vi "DrawStringOnFrontImage.vi"(6 "color(black)":u32(colorbox), 8 "error in":errorcluster, 10 "input string":string, 11 "Graph Ref":refnum<vi>) -> (0 "error out":errorcluster, 2 "picture out":picture)   [LabVIEW 2023]
doc: "Draws an Image according to input string and sets it as the Graph's front image."
uses:
  StringFormatGlobals.vi
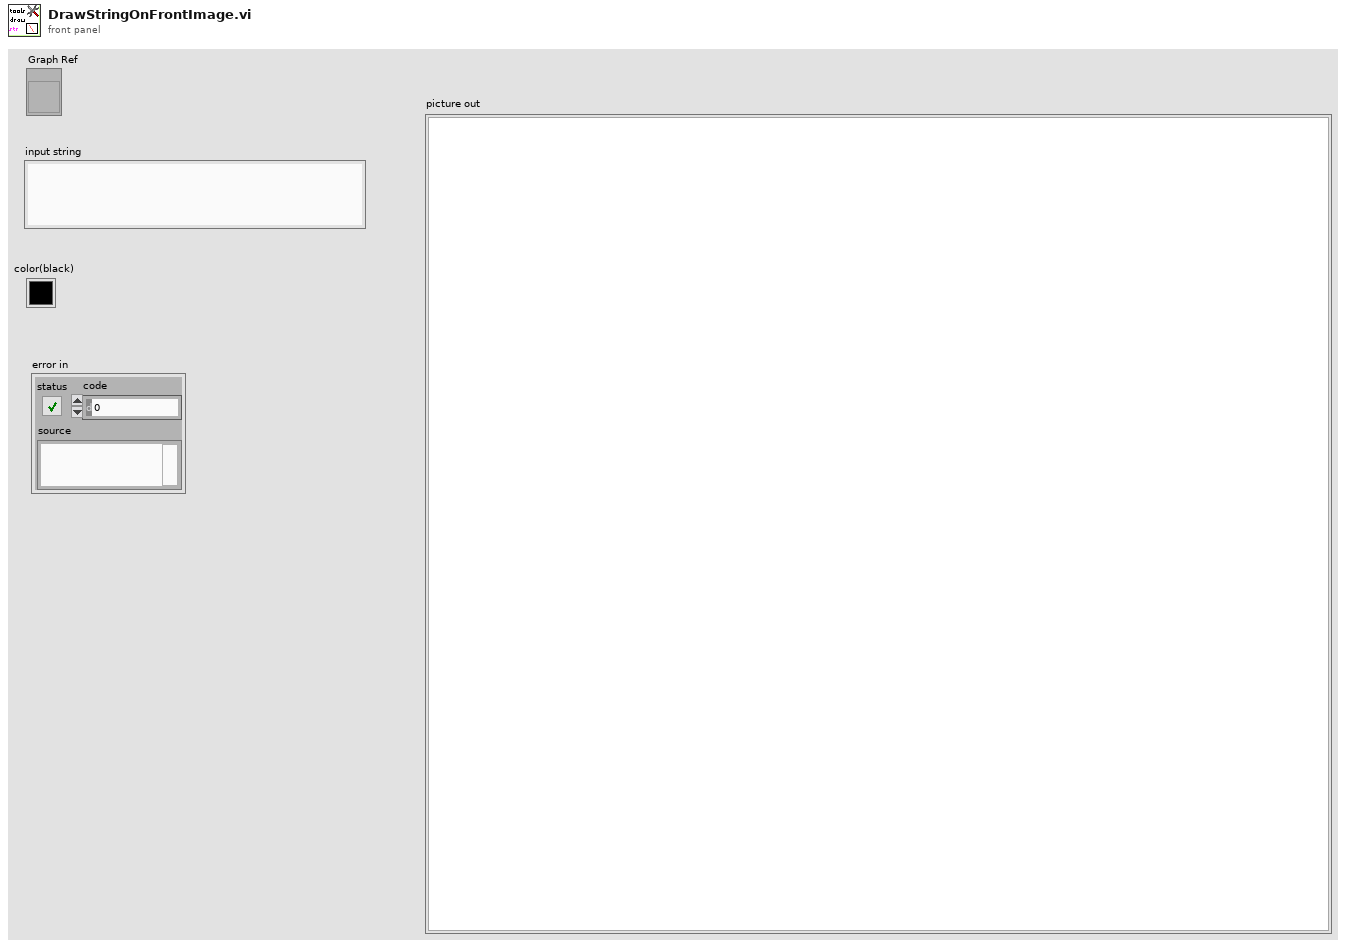
[diagram p1: front panel]
types:
  T1 = cluster{"Width":u16, "Style":enum32{"Solid", "Dash", "Dot", "DashDot", "DashDotDot"}}
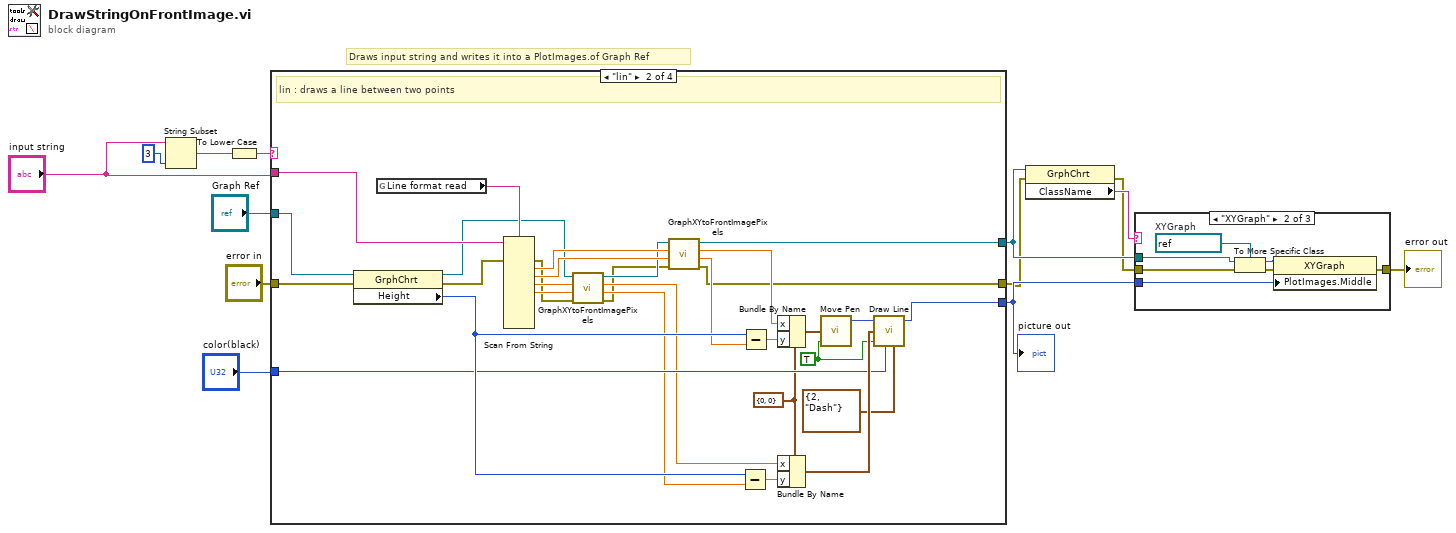
[diagram p0: block diagram]
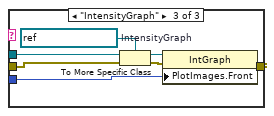
[diagram p3: hidden frame]
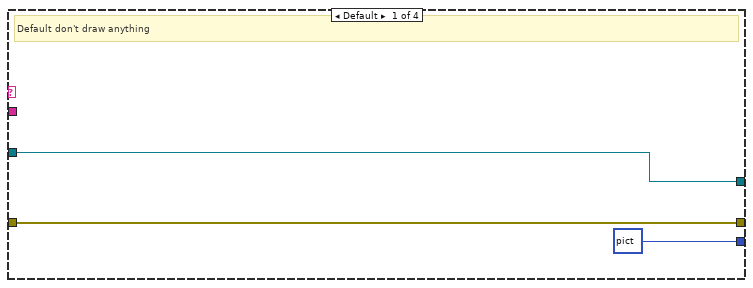
[diagram p4: hidden frame]
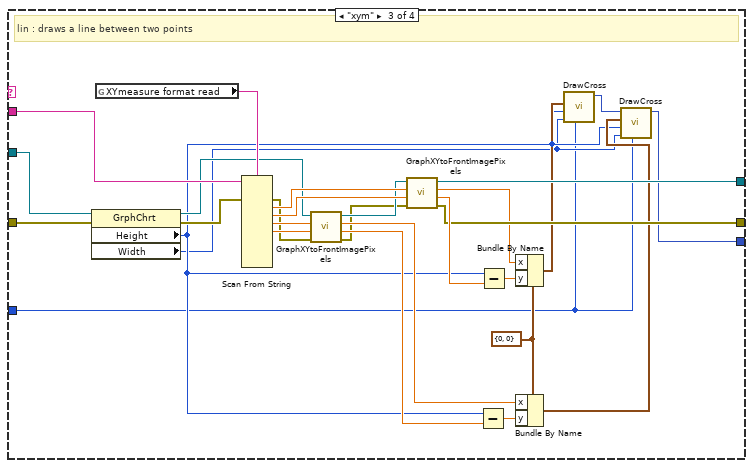
[diagram p5: hidden frame]
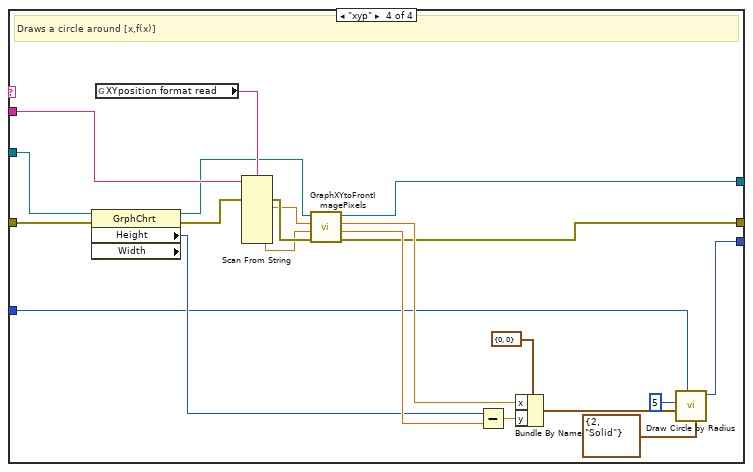
[diagram p6: hidden frame]
diagram:
  # "Draws input string and writes it into a PlotImages.of Graph Ref"
  n1 = String Subset(string="input string", length (rest)=3 ("length (rest)")) -> (substring=w2:string)  [unwired: 1 in]
  n2 = To Lower Case(string=w2) -> (all lower case string=w1:string)
  n3 = case shown="\"lin\"" w1 {
    tunnel: "input string" -> [_ w43 w75 w96]
    tunnel: [w15 w30 w68 w83] -> w7
    tunnel: [picture data[5B] ("new picture") w39 w52 w80] -> w8
    tunnel: "Graph Ref" -> [w15 w38 w73 w94]
    tunnel: "error in" -> [w14 w36 w71 w92]
    tunnel: [w14 w17 w56 w82] -> w4
    tunnel: "color(black)" -> [_ w34 w47 w79]
    frame Default {
      # "Default don't draw anything"
    }
    frame "lin" {
      w40 = TRUE ("absolute coordinates?(T)")
      w32 = cluster{"x":i16, "y":i16} {"x"=0, "y"=0} ("new position")
      # "lin : draws a line between two points"
      n4 = property on="Property Node" class="GrphChrt"(reference=w38, error in=w36) -> (reference out=w25:refnum<vi>, error out=w37:errorcluster, "Height"=w41:u32)
      n5 = global read "StringFormatGlobals.vi" "Line format read"() -> (w35:string)
      n6 = Scan From String(format string=w35, input string=w43, error in=w37) -> (error out=w19:errorcluster, output 1=w29:dbl, output 2=w28:dbl, output 3=w23:dbl, output 4=w22:dbl)  [unwired: 13 in, 2 out]
      n7 = call "GraphXYtoFrontImagePixels.vi"("error in (no error)"=w19, "Graph Y"=w22, "Graph X"=w23, "IntensityGraph in"=w25) -> ("error out"=w18:errorcluster, "Pixel Y"=w20:dbl, "Pixel X"=w21:dbl, "IntensityGraph out"=w24:refnum<vi>)  [unwired: 4 in]
      n8 = call "GraphXYtoFrontImagePixels.vi"("error in (no error)"=w18, "Graph Y"=w28, "Graph X"=w29, "IntensityGraph in"=w24) -> ("error out"=w17:errorcluster, "Pixel Y"=w27:dbl, "Pixel X"=w26:dbl, "IntensityGraph out"=w30:refnum<vi>)  [unwired: 4 in]
      n9 = Subtract(x=w41, y=w20) -> (x-y=w42:dbl)
      n10 = Subtract(x=w41, y=w27) -> (x-y=w31:dbl)
      n11 = Bundle By Name(cluster=w32, "x"=w26, "y"=w31) -> (w33:cluster{"x":i16, "y":i16})
      n12 = Bundle By Name(cluster=w32, "x"=w21, "y"=w42) -> (w45:cluster{"x":i16, "y":i16})
      n13 = call <vilib>:"Move Pen.vi"("absolute coordinates?(T)"=w40, "new position"=w33) -> ("new picture"=w46:picture)  [unwired: 3 in]
      n14 = call <vilib>:"Draw Line.vi"("picture"=w46, "end point"=w45, "absolute coordinates?(T)"=w40, "color(black)"=w34, "pen"=T1 {"Width"=2, "Style"=enum."Dash"}) -> ("new picture"=w39:picture)  [unwired: 4 in]
    }
    frame "xym" {
      w69 = cluster{"x":i16, "y":i16} {"x"=0, "y"=0} ("new position")
      # "lin : draws a line between two points"
      n15 = property on="Property Node" class="GrphChrt"(reference=w73, error in=w71) -> (reference out=w64:refnum<vi>, error out=w72:errorcluster, "Height"=w49:u32, "Width"=w48:u32)
      n16 = global read "StringFormatGlobals.vi" "XYmeasure format read"() -> (w70:string)
      n17 = Scan From String(format string=w70, input string=w75, error in=w72) -> (error out=w58:errorcluster, output 1=w67:dbl, output 2=w66:dbl, output 3=w62:dbl, output 4=w61:dbl)  [unwired: 13 in, 2 out]
      n18 = call "GraphXYtoFrontImagePixels.vi"("error in (no error)"=w58, "Graph Y"=w61, "Graph X"=w62, "IntensityGraph in"=w64) -> ("error out"=w57:errorcluster, "Pixel Y"=w59:dbl, "Pixel X"=w60:dbl, "IntensityGraph out"=w63:refnum<vi>)  [unwired: 4 in]
      n19 = call "GraphXYtoFrontImagePixels.vi"("error in (no error)"=w57, "Graph Y"=w66, "Graph X"=w67, "IntensityGraph in"=w63) -> ("error out"=w56:errorcluster, "Pixel Y"=w65:dbl, "Pixel X"=w55:dbl, "IntensityGraph out"=w68:refnum<vi>)  [unwired: 4 in]
      n20 = Subtract(x=w49, y=w59) -> (x-y=w74:dbl)
      n21 = Subtract(x=w49, y=w65) -> (x-y=w54:dbl)
      n22 = Bundle By Name(cluster=w69, "x"=w55, "y"=w54) -> (w50:cluster{"x":i16, "y":i16})
      n23 = Bundle By Name(cluster=w69, "x"=w60, "y"=w74) -> (w51:cluster{"x":i16, "y":i16})
      n24 = call "DrawCross.vi"("color(black)"=w47, "Width"=w48, "Height"=w49, "new position"=w50) -> ("new picture"=w53:picture)  [unwired: 7 in]
      n25 = call "DrawCross.vi"("color(black)"=w47, "Width"=w48, "Height"=w49, "new position"=w51, "picture"=w53) -> ("new picture"=w52:picture)  [unwired: 6 in]
    }
    frame "xyp" {
      # "Draws a circle around [x,f(x)]"
      n26 = property on="Property Node" class="GrphChrt" props=["Height", "Width"](reference=w94, error in=w92) -> (reference out=w89:refnum<vi>, error out=w93:errorcluster, "Height"=w85:u32)  [unwired: 1 out]
      n27 = global read "StringFormatGlobals.vi" "XYposition format read"() -> (w91:string)
      n28 = Scan From String(format string=w91, input string=w96, error in=w93) -> (error out=w86:errorcluster, output 1=w84:dbl, output 5=w81:dbl)  [unwired: 9 in, 2 out]
      n29 = call "GraphXYtoFrontImagePixels.vi"("error in (no error)"=w86, "Graph Y"=w81, "Graph X"=w84, "IntensityGraph in"=w89) -> ("error out"=w82:errorcluster, "Pixel Y"=w87:dbl, "Pixel X"=w88:dbl, "IntensityGraph out"=w83:refnum<vi>)  [unwired: 4 in]
      n30 = Subtract(x=w85, y=w87) -> (x-y=w95:dbl)
      n31 = Bundle By Name(cluster=cluster{"x":i16, "y":i16} {"x"=0, "y"=0} ("new position"), "x"=w88, "y"=w95) -> (w78:cluster{"x":i16, "y":i16})
      n32 = call <vilib>:"Draw Circle by Radius.vi"("pen"=T1 {"Width"=2, "Style"=enum."Solid"}, "color(black)"=w79, "pixel center"=w78, "radius"=i16 5) -> ("new picture"=w80:picture)  [unwired: 7 in]
    }
  }
  "picture out" <- w8
  n33 = property class="GrphChrt"(reference=w7, error in=w4) -> (error out=w3:errorcluster, "ClassName"=w5:string)  [unwired: 1 out]
  n34 = case shown="\"XYGraph\"" w5 {
    tunnel: w3 -> [w97 w102 w109]
    tunnel: w8 -> [_ w104 w111]
    tunnel: w7 -> [_ w101 w108]
    tunnel: [w97 w103 w110] -> w6
    frame Default {
    }
    frame "XYGraph" {
      w100 = refnum<vi> refnum  # XYGraph
      n35 = To More Specific Class(target class=w100, reference=w101, error in=w102) -> (specific class reference=w99:refnum<vi>, error out=w98:errorcluster)
      n36 = property on="Property Node" class="XYGraph"(reference=w99, error in=w98, "PlotImages.Middle"=w104) -> (error out=w103:errorcluster)  [unwired: 1 out]
    }
    frame "IntensityGraph" {
      w107 = refnum<vi> refnum  # IntensityGraph
      n37 = To More Specific Class(target class=w107, reference=w108, error in=w109) -> (specific class reference=w106:refnum<vi>, error out=w105:errorcluster)
      n38 = property on="Property Node" class="IntGraph"(reference=w106, error in=w105, "PlotImages.Front"=w111) -> (error out=w110:errorcluster)  [unwired: 1 out]
    }
  }
  "error out" <- w6
